vi "Find Block Diagram Resource.vi"(11 "Resources":T2) -> (1 "Index":i32, 2 "Found?":bool, 3 "Resource":T1)   [LabVIEW 2018, in "Resource Manipulation.lvlib"]
uses:
  Resource Manipulation.lvlib
  Resource Manipulation/Resource Array.ctl
  Resource Manipulation/Resource.ctl
  Resource Manipulation/Find First Matching Resource (String).vi
  Resource Manipulation/Find Resource by Type (String).vi
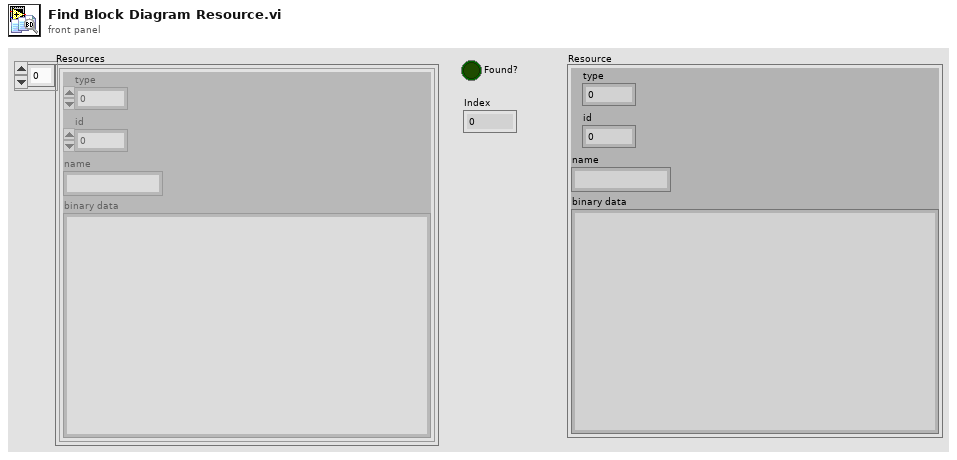
[diagram p1: front panel]
types:
  T1 = typedef "Resource Manipulation.lvlib/Resource.ctl" = cluster{"type":u32, "id":i32, "name":string, "binary data":string}
  T2 = typedef "Resource Manipulation.lvlib/Resource Array.ctl" = T1[]
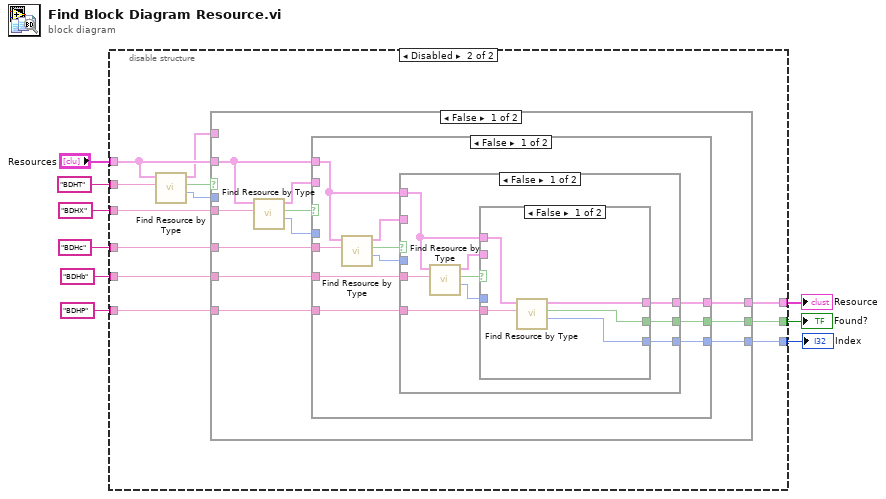
[diagram p0: block diagram]
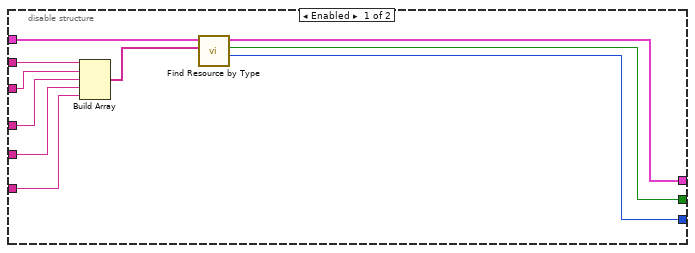
[diagram p2: hidden frame]
diagram:
  n1 = disable-structure shown="Disabled" {
    disable-tunnel: "BDHX" -> [w18 w31]
    disable-tunnel: "BDHc" -> [w17 w30]
    disable-tunnel: "BDHb" -> [w16 w29]
    disable-tunnel: "BDHP" -> [w15 w28]
    disable-tunnel: [w10 w27] -> w5
    disable-tunnel: [w12 w26] -> w4
    disable-tunnel: [w11 w25] -> w3
    disable-tunnel: "Resources" -> [w14 w24]
    disable-tunnel: "BDHT" -> [w19 w23]
    frame Enabled {
      n2 = Build Array(w19, w18, w17, w16, w15) -> (w13:string[])
      n3 = call-poly "Find Resource by Type.vi"("Resource Types"=w13, "Resources"=w14) -> ("Index"=w10:i32, "Found?"=w11:bool, "Resource"=w12:T1)  [unwired: 6 in, 1 out]
    }
    frame Disabled {
      n4 = call-poly "Find Resource by Type.vi"("Resource Type"=w23, "Resources"=w24) -> ("Index"=w20:i32, "Found?"=w22:bool, "Resource"=w21:T1)  [unwired: 6 in, 1 out]
      n5 = case shown="False" w22 {
        selector: w22 -> [_ w77]
        tunnel: w31 -> [w42 _]
        tunnel: w30 -> [w40 _]
        tunnel: w29 -> [w39 _]
        tunnel: w24 -> [w38 _]
        tunnel: w28 -> [w37 _]
        tunnel: [w36 w76] -> w27
        tunnel: [w35 w78] -> w26
        tunnel: [w34 w77] -> w25
        tunnel: w21 -> [_ w78]
        tunnel: w20 -> [_ w76]
        frame False {
          n6 = call-poly "Find Resource by Type.vi"("Resource Type"=w42, "Resources"=w38) -> ("Index"=w32:i32, "Found?"=w41:bool, "Resource"=w33:T1)  [unwired: 6 in, 1 out]
          n7 = case shown="False" w41 {
            selector: w41 -> [_ w74]
            tunnel: w40 -> [w52 _]
            tunnel: w39 -> [w50 _]
            tunnel: w38 -> [w49 _]
            tunnel: w37 -> [w48 _]
            tunnel: [w47 w75] -> w35
            tunnel: [w46 w74] -> w34
            tunnel: [w45 w73] -> w36
            tunnel: w33 -> [_ w75]
            tunnel: w32 -> [_ w73]
            frame False {
              n8 = call-poly "Find Resource by Type.vi"("Resource Type"=w52, "Resources"=w49) -> ("Index"=w43:i32, "Found?"=w51:bool, "Resource"=w44:T1)  [unwired: 6 in, 1 out]
              n9 = case shown="False" w51 {
                selector: w51 -> [_ w71]
                tunnel: w50 -> [w61 _]
                tunnel: w49 -> [w59 _]
                tunnel: w48 -> [w58 _]
                tunnel: [w57 w72] -> w47
                tunnel: [w56 w71] -> w46
                tunnel: [w55 w70] -> w45
                tunnel: w44 -> [_ w72]
                tunnel: w43 -> [_ w70]
                frame False {
                  n10 = call-poly "Find Resource by Type.vi"("Resource Type"=w61, "Resources"=w59) -> ("Index"=w53:i32, "Found?"=w60:bool, "Resource"=w54:T1)  [unwired: 6 in, 1 out]
                  n11 = case shown="False" w60 {
                    selector: w60 -> [_ w67]
                    tunnel: w59 -> [w66 _]
                    tunnel: w58 -> [w65 _]
                    tunnel: [w64 w69] -> w57
                    tunnel: [w63 w67] -> w56
                    tunnel: [w62 w68] -> w55
                    tunnel: w54 -> [_ w69]
                    tunnel: w53 -> [_ w68]
                    frame False {
                      n12 = call-poly "Find Resource by Type.vi"("Resource Type"=w65, "Resources"=w66) -> ("Index"=w62:i32, "Found?"=w63:bool, "Resource"=w64:T1)  [unwired: 6 in, 1 out]
                    }
                    frame True {
                    }
                  }
                }
                frame True {
                }
              }
            }
            frame True {
            }
          }
        }
        frame True {
        }
      }
    }
  }
  "Resource" <- w4
  "Found?" <- w3
  "Index" <- w5
